vi "Read and Write Controls to Config File.vi"(5 "section (optional)":string, 7 "Action":T1, 8 "error in":errorcluster, 10 "Control References":refnum<vi>[](array[refnum]), 11 "Configuration File Reference In":T2) -> (0 "error out":errorcluster, 3 "Configuration File Reference Out":T2)   [LabVIEW 2021]
doc: "Writes the values of an array of controls to a configuration file or reads them back.\n<b>Control References</b> is an array of the references of the controls to be saved.\n\nThe section name is the name of the VI that holds the control.\nThe key name is the label of the control."
uses:
  <vilib>/Utility/config.llb/Config Data RefNum.ctl
  RWC_Actions.ctl
  <vilib>/Utility/config.llb/Read Key (String).vi
  <vilib>/Utility/config.llb/Write Key (String).vi
  <vilib>/Utility/config.llb/NI_LVConfig.lvlib
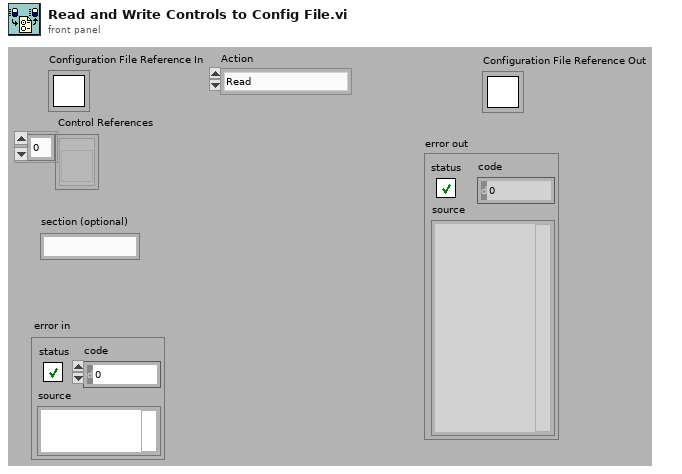
[diagram p1: front panel]
types:
  T1 = typedef "RWC_Actions.ctl" = enum16{"Read", "Write", "Read and Create"}
  T2 = typedef "NI_LVConfig.lvlib/Config Data RefNum.ctl" = refnum<k1>
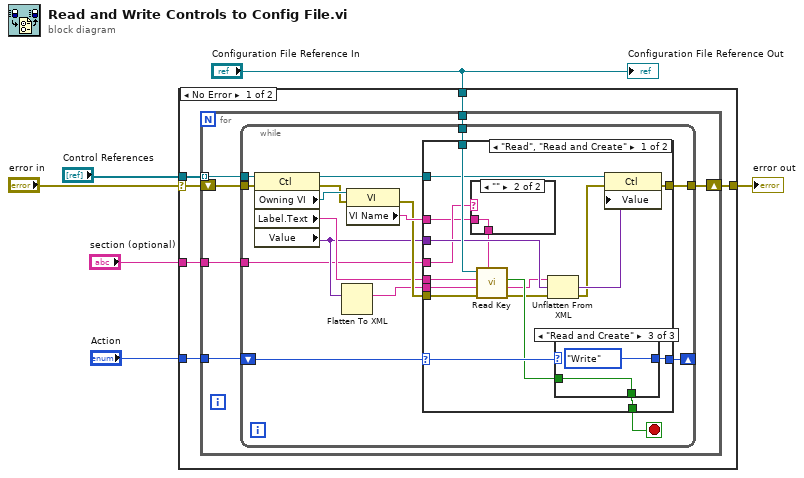
[diagram p0: block diagram]
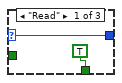
[diagram p3: hidden frame]
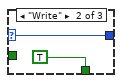
[diagram p4: hidden frame]
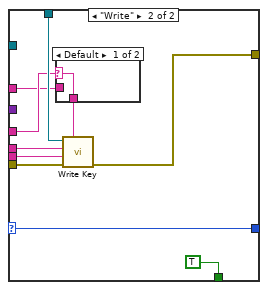
[diagram p5: hidden frame]
diagram:
  n1 = case shown="No Error" "error in" {
    selector: "error in" -> [w9 w73]
    tunnel: "Control References" -> [w12 _]
    tunnel: [w11 w73] -> w5
    tunnel: "Configuration File Reference In" -> [w10 _]
    tunnel: "Action" -> [w8 _]
    tunnel: "section (optional)" -> [w7 _]
    frame No Error {
      n2 = for {
        tunnel: w12 -> [w18] mode=indexing
        shift-right: [w16] -> w11
        shift-left: w9 -> [w17]
        tunnel: w10 -> [w15]
        tunnel: w8 -> [w14]
        tunnel: w7 -> [w13]
        n3 = while {
          tunnel: w18 -> [w34]
          tunnel: w17 -> [w33]
          tunnel: [w32] -> w16
          tunnel: w15 -> [w31]
          shift-right: [w23] -> _
          shift-left: w14 -> [w24]
          tunnel: w13 -> [w19]
          stop <- w25 stop-if-true
          n4 = property class="Ctl"(reference=w34, error in=w33) -> (reference out=w26:refnum<vi>, error out=w28:errorcluster, "Owning VI"=w30:refnum<vi>, "Label.Text"=w22:string, "Value"=w21:variant)
          n5 = Flatten To XML(6:w21) -> (2:w20:string)
          n6 = property class="VI"(reference=w30, error in=w28) -> (error out=w27:errorcluster, "VI Name"=w29:string)  [unwired: 1 out]
          n7 = case shown="\"Read\", \"Read and Create\"" w24 {
            selector: w24 -> [w47 w65]
            tunnel: [w48 w70] -> w32
            tunnel: w31 -> [w50 w69]
            tunnel: w29 -> [w36 w62]
            tunnel: w22 -> [w51 w68]
            tunnel: w27 -> [w52 w67]
            tunnel: w26 -> [w49 _]
            tunnel: [w46 TRUE] -> w25
            tunnel: [w45 w65] -> w23
            tunnel: w20 -> [w43 w64]
            tunnel: w21 -> [w42 _]
            tunnel: w19 -> [w37 w63]
            frame "Read", "Read and Create" {
              n8 = case shown="\"\"" w37 {
                selector: w37 -> [w53 _]
                tunnel: [w53 w54] -> w35
                tunnel: w36 -> [_ w54]
                frame Default {
                }
                frame "" {
                }
              }
              n9 = call-poly <vilib>:"Read Key.vi"("section"=w35, "error in (no error)"=w52, "default value"=w43, "key"=w51, "refnum"=w50) -> ("error out"=w38:errorcluster, "value"=w41:string, "found?"=w44:bool)  [unwired: 3 in, 1 out]
              n10 = Unflatten From XML(xml string=w41, type=w42, error in (no error)=w38) -> (value=w40:variant, error out=w39:errorcluster)
              n11 = case shown="\"Read and Create\"" w47 {
                selector: w47 -> [w56 w57 _]
                tunnel: [TRUE ("found?") TRUE w60] -> w46
                tunnel: [w56 w57 RWC_Actions."Write"] -> w45
                tunnel: w44 -> [_ _ w60]
                frame "Read" {
                }
                frame "Write" {
                }
                frame "Read and Create" {
                }
              }
              n12 = property class="Ctl"(reference=w49, error in=w39, "Value"=w40) -> (error out=w48:errorcluster)  [unwired: 1 out]
            }
            frame "Write" {
              n13 = case shown="Default" w63 {
                selector: w63 -> [w71 _]
                tunnel: [w71 w72] -> w61
                tunnel: w62 -> [_ w72]
                frame Default {
                }
                frame "" {
                }
              }
              n14 = call-poly <vilib>:"Write Key.vi"("section"=w61, "error in (no error)"=w67, "value"=w64, "key"=w68, "refnum"=w69) -> ("error out"=w70:errorcluster)  [unwired: 4 in, 2 out]
            }
          }
        }
      }
    }
    frame Error {
    }
  }
  "error out" <- w5
  "Configuration File Reference Out" <- "Configuration File Reference In"
